vi "NC_varoffset.vi"(4 "coord":u64[](array[numeric]), 5 "NC_var":T1 {"NC_attrarray"."nc_type" items=["NC_NAT", "NC_BYTE", "NC_CHAR", "NC_SHORT", "NC_INT", "NC_FLOAT", "NC_DOUBLE"]}) -> (0 "lcoord":u64)   [LabVIEW 2016]
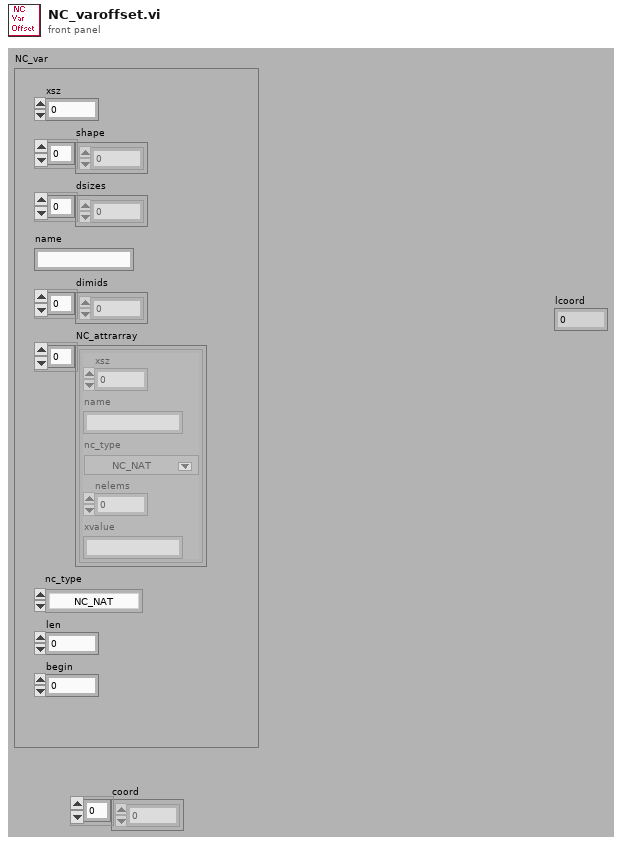
[diagram p1: front panel]
types:
  T1 = cluster{"xsz":u64, "shape":u64[], "dsizes":u64[], "name":string, "dimids":u64[], "NC_attrarray":cluster{"xsz":u64, "name":string, "nc_type":u16, "nelems":u64, "xvalue":string}[], "nc_type":enum16{"NC_NAT", "NC_BYTE", "NC_CHAR", "NC_SHORT", "NC_INT", "NC_FLOAT", "NC_DOUBLE"}, "len":u64, "begin":u64}
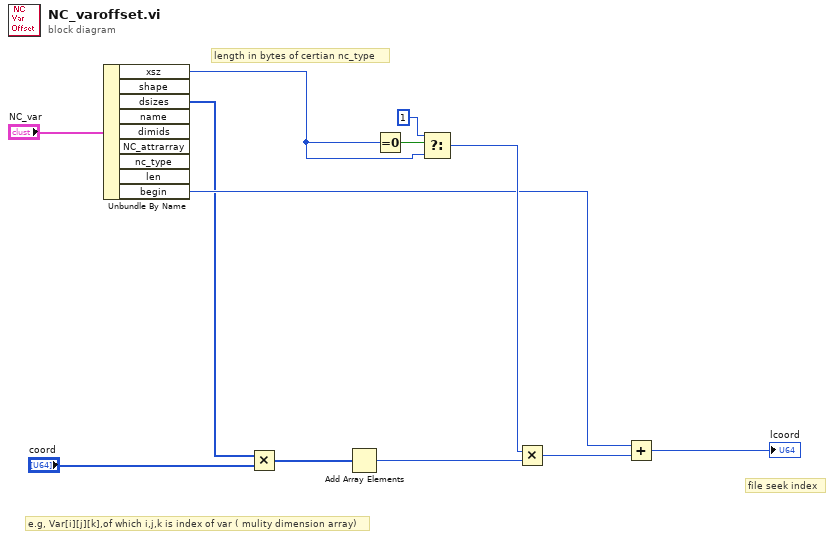
[diagram p0: block diagram]
diagram:
  # "file seek index"
  # "length in bytes of certian nc_type"
  # "e.g, Var[i][j][k],of which i,j,k is index of var ( mulity dimension array)"
  n1 = Unbundle By Name("NC_var") -> ("xsz"=w5:u64, "dsizes"=w4:u64[], "begin"=w6:u64)  [unwired: 6 out]
  n2 = Multiply(x=w4, y="coord") -> (x*y=w2:u64[])
  n3 = Add Array Elements(numeric array=w2) -> (sum=w1:u64)
  n4 = Equal To 0?(x=w5) -> (x = 0?=w12:bool)
  n5 = Select(t=u64 1, s=w12, f=w5) -> (s? t:f=w10:u64)
  n6 = Multiply(x=w10, y=w1) -> (x*y=w9:u64)
  n7 = Add(x=w6, y=w9) -> (x+y=→"lcoord":u64)
